vi "Spreadsheet Read.vi"() -> ()   [LabVIEW 2017]
panel:
  out "XY Graph":cluster{dbl[], dbl[]}(graph)
  out "subarray 2":dbl[](array[numeric])
  out "subarray":dbl[](array[numeric])
  out "Output Cluster":cluster{"X Array":dbl[], "Y Array":dbl[]}
  out "array":dbl[][](array[numeric])
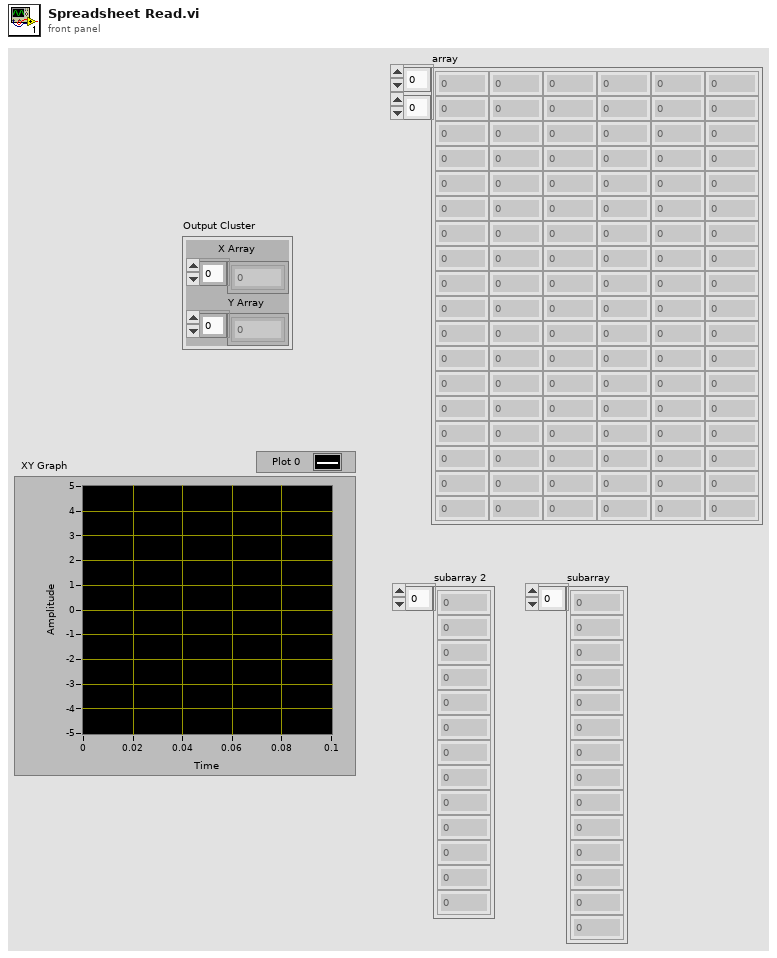
[diagram p1: front panel]
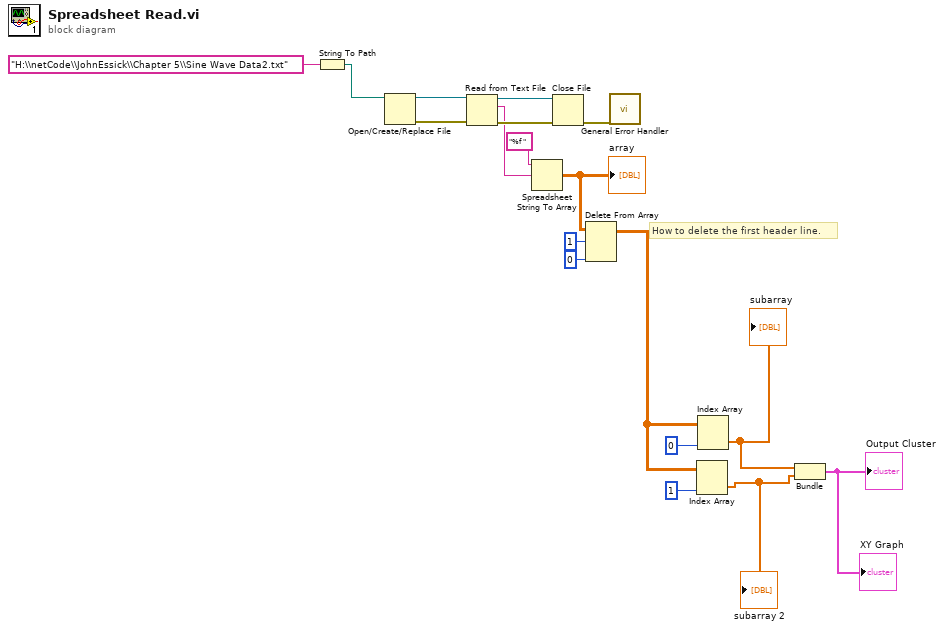
[diagram p0: block diagram]
diagram:
  # "How to delete the first header line."
  n1 = String To Path(string="H:\\netCode\\JohnEssick\\Chapter 5\\Sine Wave Data2.txt") -> (path=w17:path)
  n2 = Open/Create/Replace File(file path (use dialog)=w17) -> (refnum out=w16:refnum<file>, error out=w14:errorcluster)  [unwired: 5 in, 1 out]
  n3 = Read from Text File(file (use dialog)=w16, error in=w14) -> (refnum out=w15:refnum<file>, text=w11:string, error out=w13:errorcluster)  [unwired: 2 in, 1 out]
  n4 = Spreadsheet String To Array(format string="%f ", spreadsheet string=w11) -> (array=w7:dbl[][])  [unwired: 2 in]
  "array" <- w7
  n5 = Close File(refnum=w15, error in=w13) -> (error out=w12:errorcluster)  [unwired: 1 out]
  n6 = Delete From Array "Delete From Array"(array=w7, length=1, index (row)=0) -> (array with subset deleted=w4:dbl[][])  [unwired: 1 in, 1 out]
  n7 = call <vilib>:"General Error Handler.vi"("error in (no error)"=w12) -> ()  [unwired: 10 in, 5 out]
  n8 = Index Array(array=w4, index (col)=1) -> (element=w2:dbl[])  [unwired: 1 in]
  "subarray 2" <- w2
  n9 = Index Array "Index Array"(array=w4, index (col)=0) -> (element=w3:dbl[])  [unwired: 1 in]
  "subarray" <- w3
  n10 = Bundle "Bundle"(w3, w2) -> (→"Output Cluster" →"XY Graph":cluster{dbl[], dbl[]})  [unwired: 1 in]
